vi "Refresh Module.vi"(6 "TreeControl in":refnum<vi>, 7 "Data Cluster In":T1={"Project"=refnum, "Current Selection"={"Library"=refnum, "VI"=refnum}, "Module ID"=-1, "Tree Selection"=""}, 8 "error in":errorcluster) -> (0 "error out":errorcluster, 5 "Data Cluster Out":T1={"Project"=refnum, "Current Selection"={"Library"=refnum, "VI"=refnum}, "Module ID"=-1, "Tree Selection"=""})   [LabVIEW 2020, in "Panther Dashboard.lvlib"]
doc: "Gets the Singleton and Cloneable references and creates a list of each type of DQMH Modules"
uses:
  Panther Dashboard.lvlib
  Module Data--cluster.ctl
  Class/Project/Project.lvclass
  Class/Library/Library.lvclass
  C:/GitClones/PantherDashboard/src/LabVIEW/Panther Dashboard/Class/LabVIEWItem/LabVIEWItem.lvclass
  Class/VI/VI.lvclass
  Class/Project/Project.lvclass/Project.ctl
  Class/LabVIEWItem/LabVIEWItem.lvclass/LabVIEWItem.ctl
  Class/LabVIEWItem/Item Type--enum.ctl
  Class/Library/Library.lvclass/Library.ctl
  Class/Library/Write VIs MAP.vi
  Class/LabVIEWItem/Read Item Tag.vi
  Class/Project/Write Libraries.vi
  Class/Project/Read Main App Inst Ref.vi
  Class/Project/Read Libraries.vi
  Class/LabVIEWItem/LabVIEWItem.lvclass
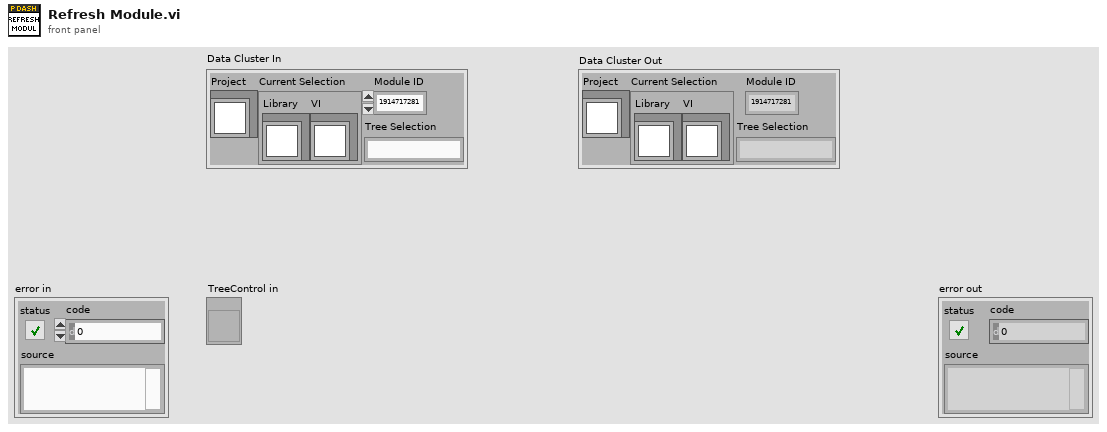
[diagram p1: front panel]
types:
  T1 = typedef "Panther Dashboard.lvlib/Module Data--cluster.ctl" = cluster{"Project":refnum<class "Project.lvclass">, "Current Selection":cluster{"Library":refnum<class "Library.lvclass">, "VI":refnum<class "VI.lvclass">}, "Module ID":i32, "Tree Selection":string}
  T2 = typedef "Panther Dashboard.lvlib/LabVIEWItem.lvclass/Item Type--enum.ctl" = enum16{"Requests", "Broadcasts", "Request and Wait for Reply", "Round Trip", "» Public API VIs", "» Constant VIs", "» Error VIs", "Module", "Project", "No Drag Selection"}
  T3 = typedef "Tree Map.lvlib/Tree Map Data.ctl" = map{string, cluster{"Child Paths Set":set{string}, "Name":string, "Data":string, "Attributes":map{string, string}}}
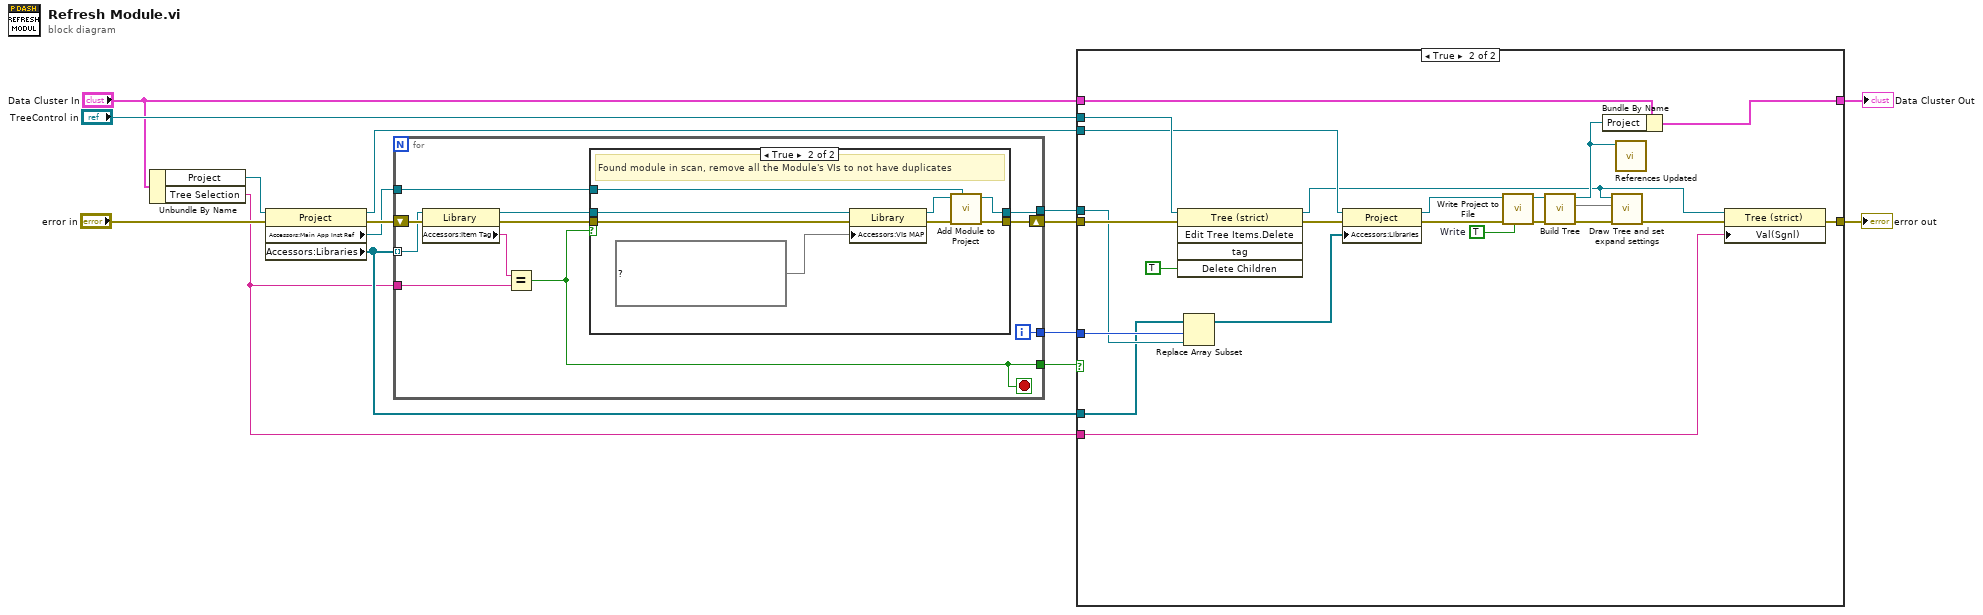
[diagram p0: block diagram]
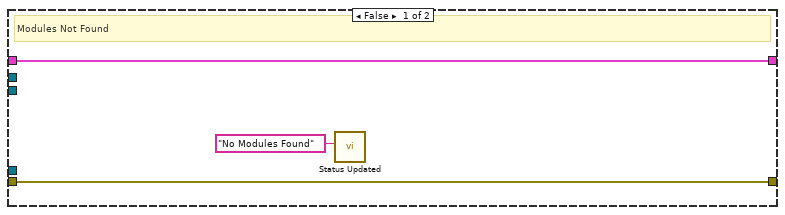
[diagram p2: hidden frame]
diagram:
  n1 = Unbundle By Name("Data Cluster In") -> ("Project"=w8:refnum<class "Project.lvclass">, "Tree Selection"=w1:string)
  n2 = property class="Project"(reference=w8, error in="error in") -> (reference out=w7:refnum<class "Project.lvclass">, error out=w15:errorcluster, "Accessors:Main App Inst Ref"=w3:refnum<vi>, "Accessors:Libraries"=w4:refnum<class "Library.lvclass">[])
  n3 = for {
    tunnel: w4 -> [w23] mode=indexing
    tunnel: w1 -> [w22]
    tunnel: [w21] -> w6
    shift-right: [w24] -> w13
    shift-left: w15 -> [w26]
    tunnel: [w18] -> w5
    tunnel: w3 -> [w19]
    tunnel: [w16] -> w2
    i -> [w21]
    stop <- w16 stop-if-true
    n4 = property class="Library"(reference=w23, error in=w26) -> (reference out=w20:refnum<class "Library.lvclass">, error out=w25:errorcluster, "Accessors:Item Tag"=w17:string)
    n5 = Equal?(x=w17, y=w22) -> (x = y?=w16:bool)
    n6 = case shown="True" w16 {
      tunnel: w25 -> [w28 w36]
      tunnel: [w28 w35] -> w24
      tunnel: w20 -> [w27 w31]
      tunnel: w19 -> [_ w33]
      tunnel: [w27 w32] -> w18
      frame False {
        # "Current module has different Tag"
      }
      frame True {
        # "Found module in scan, remove all the Module's VIs to not have duplicates"
        n7 = property class="Library"(reference=w31, error in=w36, "Accessors:VIs MAP"=map{T2, refnum<class "VI.lvclass">[]} {} ("VIs MAP")) -> (reference out=w30:refnum<class "Library.lvclass">, error out=w34:errorcluster)
        n8 = call "Add Module to Project.vi"("App Ref"=w33, "error in"=w34, "Library In"=w30) -> ("error out"=w35:errorcluster, "Library Out"=w32:refnum<class "Library.lvclass">)  [unwired: 7 in]
      }
    }
  }
  n9 = case shown="True" w2 {
    tunnel: w13 -> [w39 w62]
    tunnel: [w39 w59] -> w12
    tunnel: "TreeControl in" -> [_ w55]
    tunnel: "Data Cluster In" -> [w38 w52]
    tunnel: [w38 w51] -> w9
    tunnel: w7 -> [_ w50]
    tunnel: w6 -> [_ w45]
    tunnel: w5 -> [_ w44]
    tunnel: w4 -> [_ w41]
    tunnel: w1 -> [_ w40]
    frame False {
      # "Modules Not Found"
      n10 = call "Status Updated.vi"("Status"="No Modules Found") -> ()  [unwired: 10 in, 1 out]
    }
    frame True {
      w53 = TRUE  # Write
      n11 = invoke class="Tree (strict)" method="Edit Tree Items.Delete"(reference=w55, error in=w62, "Delete Children"=TRUE ("Delete Children?")) -> (reference out=w43:refnum<vi>, error out=w61:errorcluster)  [unwired: 2 in, 3 out]
      n12 = Replace Array Subset(array=w41, new element=w44, index=w45) -> (w42:refnum<class "Library.lvclass">[])
      n13 = property class="Project"(reference=w50, error in=w61, "Accessors:Libraries"=w42) -> (reference out=w47:refnum<class "Project.lvclass">, error out=w58:errorcluster)
      n14 = call "Write Project to File.vi"("Write"=w53, "error in"=w58, "Project In"=w47) -> ("error out"=w57:errorcluster, "Project Out"=w46:refnum<class "Project.lvclass">)  [unwired: 6 in, 1 out]
      n15 = call "Build Tree.vi"("error in"=w57, "Project in"=w46) -> ("error out"=w60:errorcluster, "Tree Map Out"=w49:T3, "Project Out"=w48:refnum<class "Project.lvclass">)  [unwired: 7 in]
      n16 = Bundle By Name(cluster=w52, "Project"=w48) -> (w51:T1)
      n17 = call "Draw Tree and set expand settings.vi"("error in"=w60, "Tree Map In"=w49, "TreeControl in"=w43) -> ("error out"=w56:errorcluster)  [unwired: 8 in]
      n18 = call "References Updated.vi"("Project"=w48) -> ()  [unwired: 10 in, 1 out]
      n19 = property class="Tree (strict)"(reference=w43, error in=w56, "Val(Sgnl)"=w40) -> (error out=w59:errorcluster)  [unwired: 1 out]
    }
  }
  "error out" <- w12
  "Data Cluster Out" <- w9
